vi "Numeric.vi"() -> ()   [LabVIEW 2022 SP3]
panel:
  in  "Numeric":dbl=1.1123 format="%#_18g"
  out "x + y":u8
  in  "y":u16
  in  "x":i16
  # "+"
  # "="
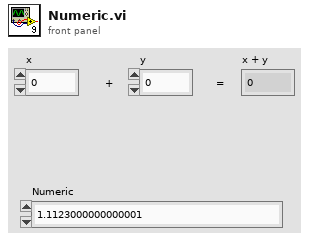
[diagram p1: front panel]
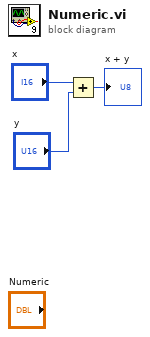
[diagram p0: block diagram]
diagram:
  n1 = Add(x="x", y="y") -> (x+y=→"x + y":u16)
